vi "SendRudderCMD.vi"(2 "error in (no error)":errorcluster, 3 "RightRudder":i32, 4 "LeftRudder":i32, 5 "Notifiers":T1) -> (0 "error out":errorcluster)   [LabVIEW 2012]
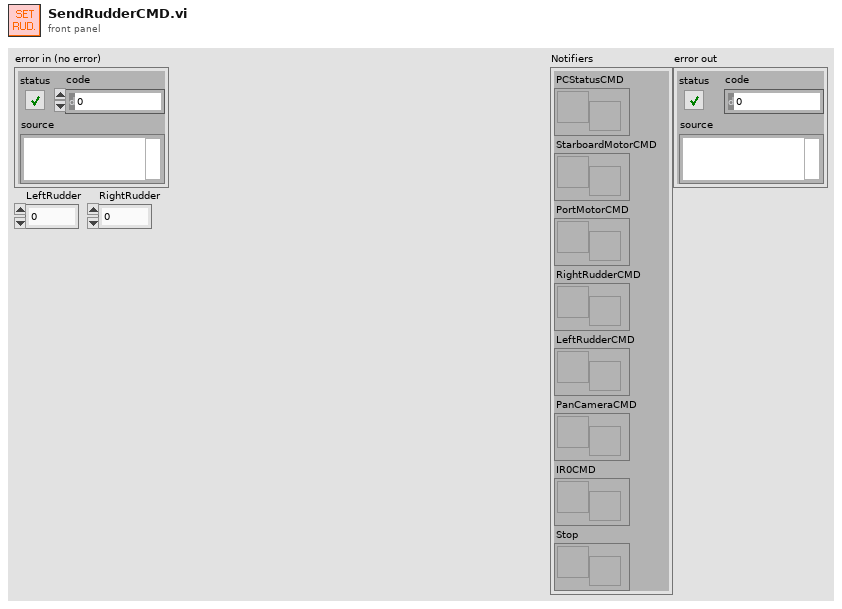
[diagram p1: front panel]
types:
  T1 = cluster{"PCStatusCMD":refnum<notifier>, "StarboardMotorCMD":refnum<notifier>, "PortMotorCMD":refnum<notifier>, "RightRudderCMD":refnum<notifier>, "LeftRudderCMD":refnum<notifier>, "PanCameraCMD":refnum<notifier>, "IR0CMD":refnum<notifier>, "Stop":refnum<notifier>}
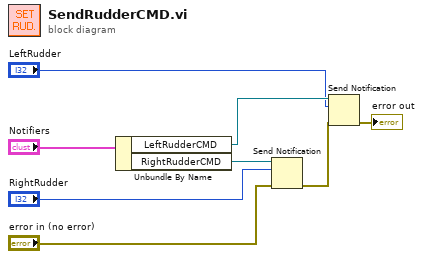
[diagram p0: block diagram]
diagram:
  n1 = Unbundle By Name("Notifiers") -> ("LeftRudderCMD"=w7:refnum<notifier>, "RightRudderCMD"=w6:refnum<notifier>)
  n2 = Send Notification(notification="RightRudder", notifier=w6, error in (no error)="error in (no error)") -> (error out=w4:errorcluster)  [unwired: 1 out]
  n3 = Send Notification(notification="LeftRudder", notifier=w7, error in (no error)=w4) -> (error out=→"error out":errorcluster)  [unwired: 1 out]
